vi "Controller.vi"() -> ()   [LabVIEW 2017]
uses:
  <vilib>/Analysis/Matrix/Datatypes/RealMatrix.ctl
  Controls/Force Torque Vector.ctl
  Controls/State.ctl
  Controls/Platform Vectors.ctl
  Controls/Constants.ctl
  Controls/Motor Position.ctl
  <vilib>/Analysis/baseanly.llb/A x Vector.vi
  <vilib>/DAQmx/read.llb/DAQmx Read (Analog 2D DBL NChan NSamp).vi
  <vilib>/Analysis/baseanly.llb/Mean (DBL).vi
  <vilib>/Analysis/baseanly.llb/Real A x B.vi
  <vilib>/Analysis/_algsub.llb/Vector Norm.vi
  <vilib>/Analysis/_algsub.llb/Real Vector Norm.vi
  <vilib>/Analysis/baseanly.llb/Outer Product.vi
  <vilib>/Analysis/baseanly.llb/Real Outer Product.vi
  <vilib>/robotics/Kinematics/Create Lie Group Matrix.vi
  <vilib>/Analysis/7linalg.llb/Create Special Real Matrix.vi
  <vilib>/Analysis/Matrix/Numeric/Multiply/Multiply.vi
  <vilib>/Analysis/Matrix/Numeric/Multiply/Multiply - RM,R.vi
  <vilib>/Analysis/Matrix/Numeric/Multiply/Multiply - R,RM.vi
  <vilib>/Analysis/Matrix/Numeric/Add/Add.vi
  <vilib>/Analysis/Matrix/Numeric/Add/Add - RM,RM.vi
  <vilib>/DAQmx/create/channels.llb/DAQmx Create Channel (AI-Voltage-Basic).vi
  <vilib>/DAQmx/configure/timing.llb/DAQmx Timing (Sample Clock).vi
  <vilib>/DAQmx/miscellaneous.llb/DAQmx Fill In Error Info.vi
  <vilib>/Analysis/3filter.llb/Butterworth Filter (DBL).vi
  <vilib>/Analysis/NI_AALBase.lvlib
  <vilib>/robotics/Kinematics/NI_Kinematics.lvlib
  <vilib>/Analysis/NI_AALPro.lvlib
  <vilib>/Analysis/Matrix/NI_Matrix.lvlib
panel:
  in  "Motor Position":T1
  in  "eta3":dbl=240.0
  in  "eta2":dbl=120.0
  in  "eta1":dbl
  out "dt":dbl=0.017
  in  "gamma2":dbl=72.0
  in  "gamma1":dbl=90.0
  in  "alpha2":dbl=90.0
  in  "alpha1":dbl=90.0
  in  "Constants":T2
  in  "Platform Vectors":T3
  in  "radius":dbl=10.0
  in  "State":T4={"Inertia"=0.5, "Damping"=1.5, "RoM"=0.0}
  out "Waveform Chart":cluster{"Fx":dbl, "Fy":dbl, "Tz":dbl}(graph)={"Fx"=16.845737208367353, "Fy"=-1.0246455882392524, "Tz"=10.011940623114288}
  in  "Force Torque Vector":T5
  in  "Calibration Matrix":T6=[[0.70287, 0.28046, -1.06379, -47.58271, -1.64459, 46.90249], [-0.12905, 55.12684, -1.23322, -27.09022, 0.94146, -27.44249], [69.23154, 1.17633, 67.18151, 0.05352, 69.14468, -0.82584], [0.02366, 0.38743, -1.10802, -0.19684, 1.1351, -0.20033], [1.26658, 0.02633, -0.60731, 0.32903, -0.6386, -0.32248], [0.02624, -0.70869, -0.00313, -0.69424, -0.02408, -0.68399]]
  in  "stop":bool
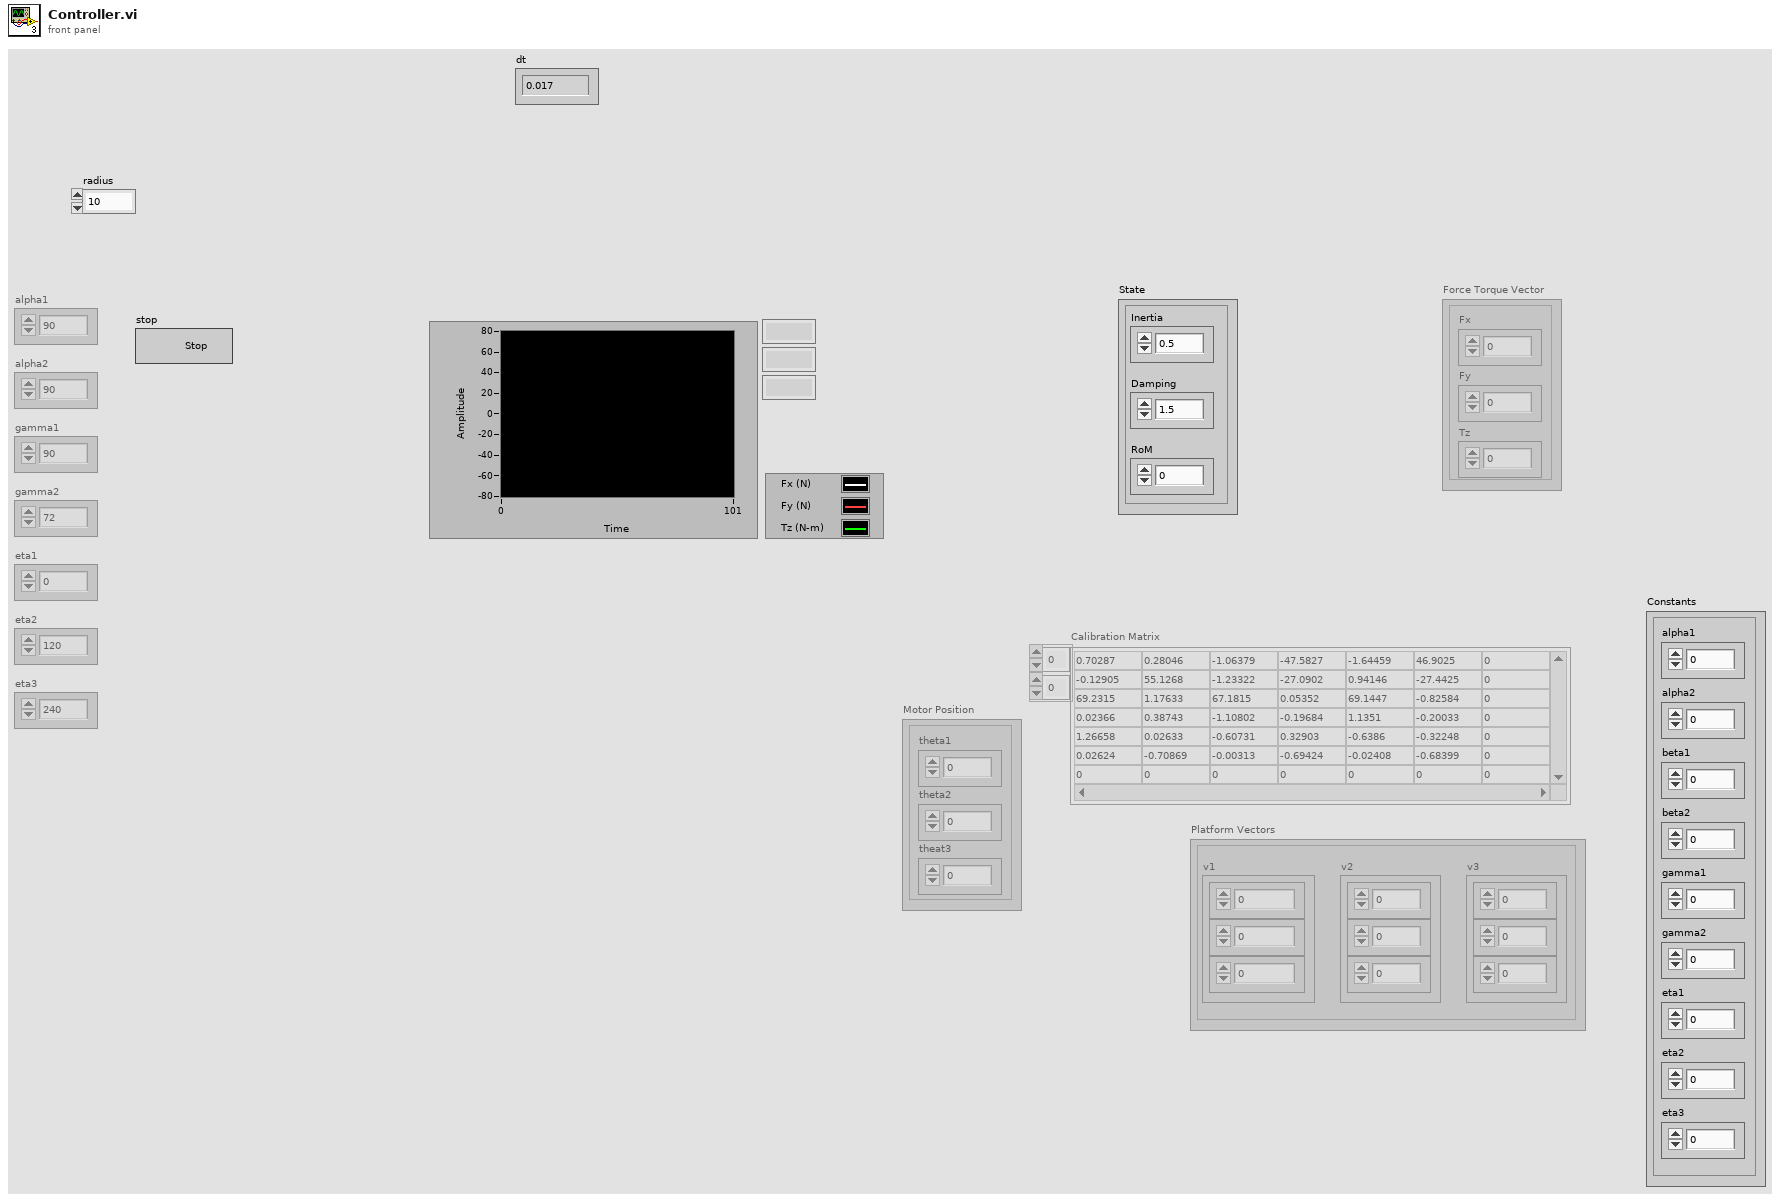
[diagram p1: front panel]
types:
  T1 = typedef "Motor Position.ctl" = cluster{"theta1":dbl, "theta2":dbl, "theat3":dbl}
  T2 = typedef "Constants.ctl" = cluster{"alpha1":dbl, "alpha2":dbl, "beta1":dbl, "beta2":dbl, "gamma1":dbl, "gamma2":dbl, "eta1":dbl, "eta2":dbl, "eta3":dbl}
  T3 = typedef "Platform Vectors.ctl" = cluster{"v1":dbl[], "v2":dbl[], "v3":dbl[]}
  T4 = typedef "State.ctl" = cluster{"Inertia":dbl, "Damping":dbl, "RoM":dbl}
  T5 = typedef "Force Torque Vector.ctl" = cluster{"Fx":dbl, "Fy":dbl, "Tz":dbl}
  T6 = typedef "NI_Matrix.lvlib/RealMatrix.ctl" = dbl[][]
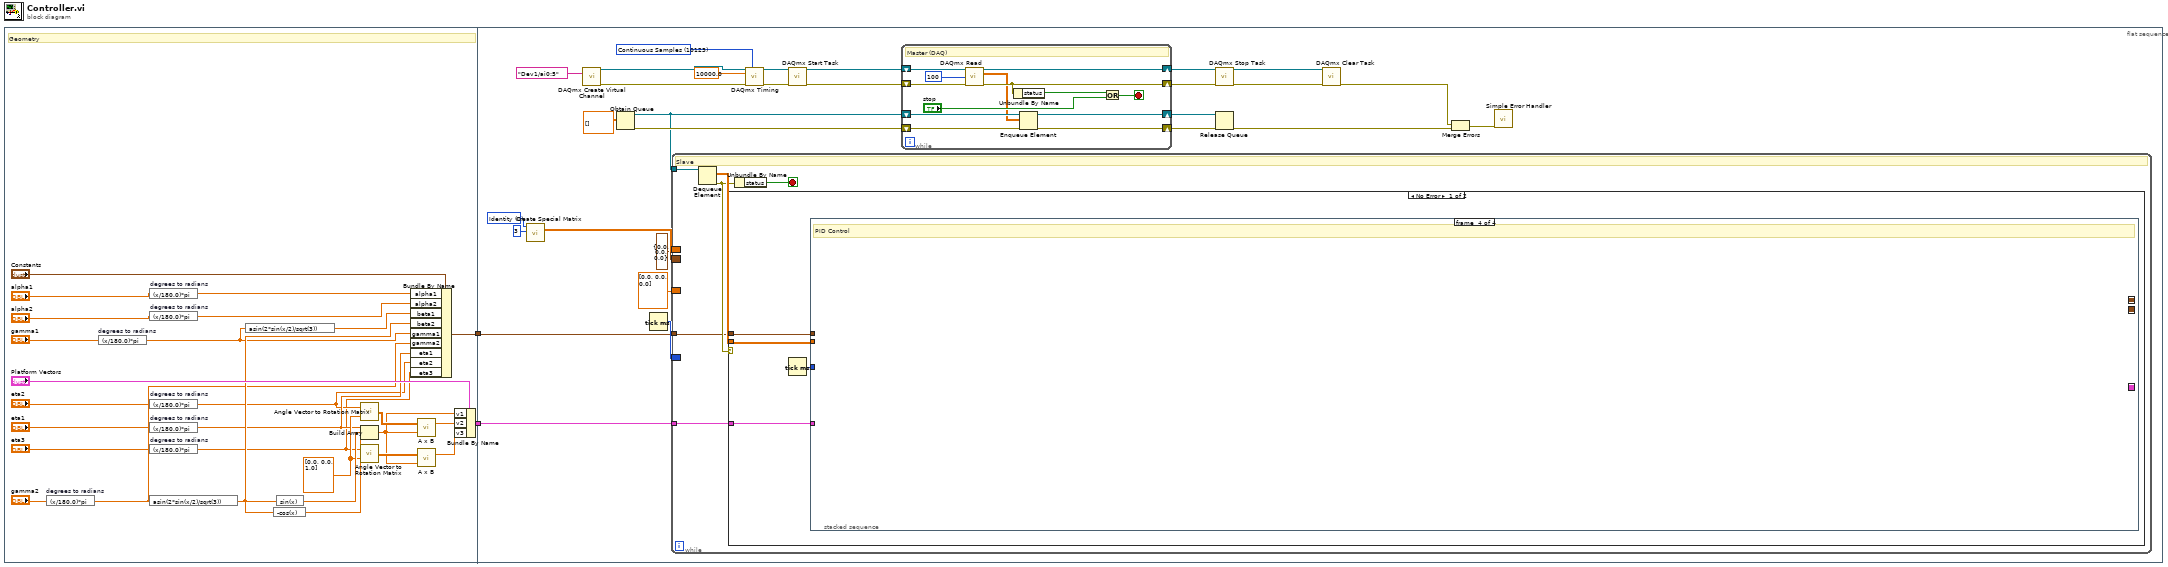
[diagram p0: block diagram]
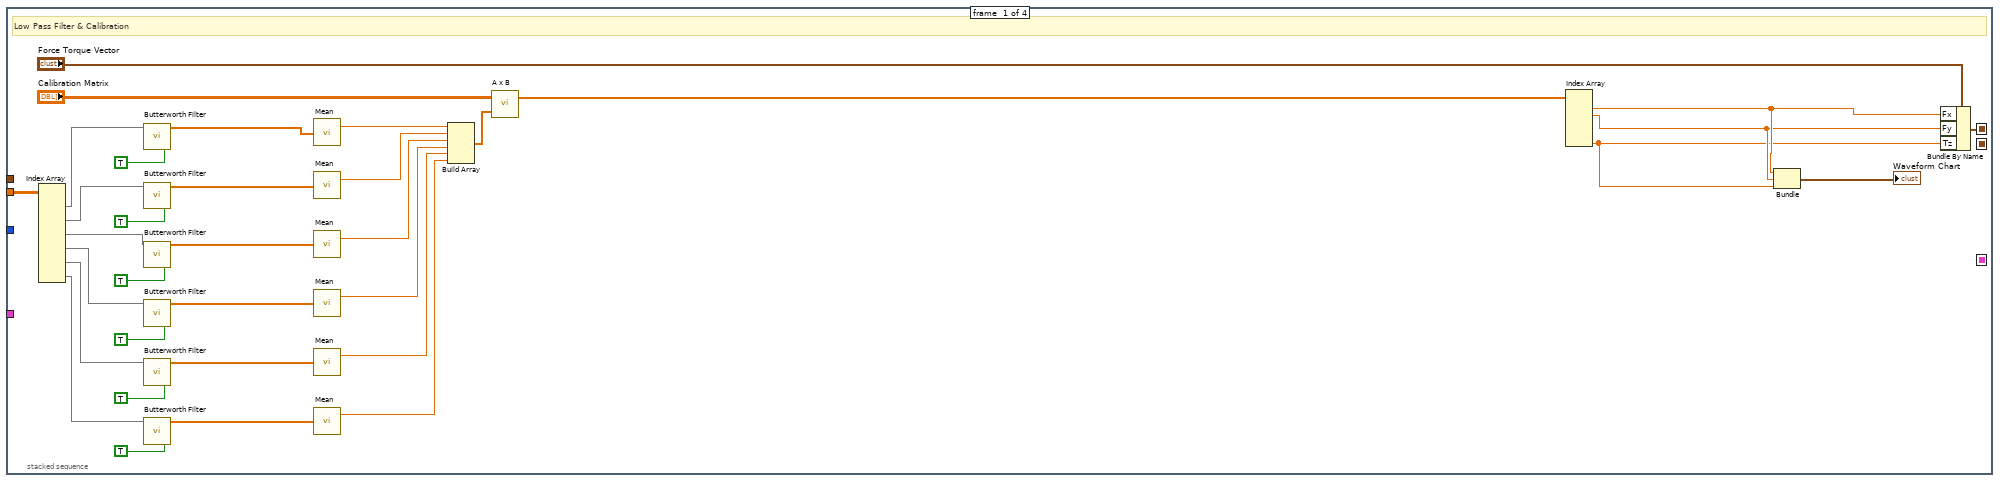
[diagram p2: hidden frame]
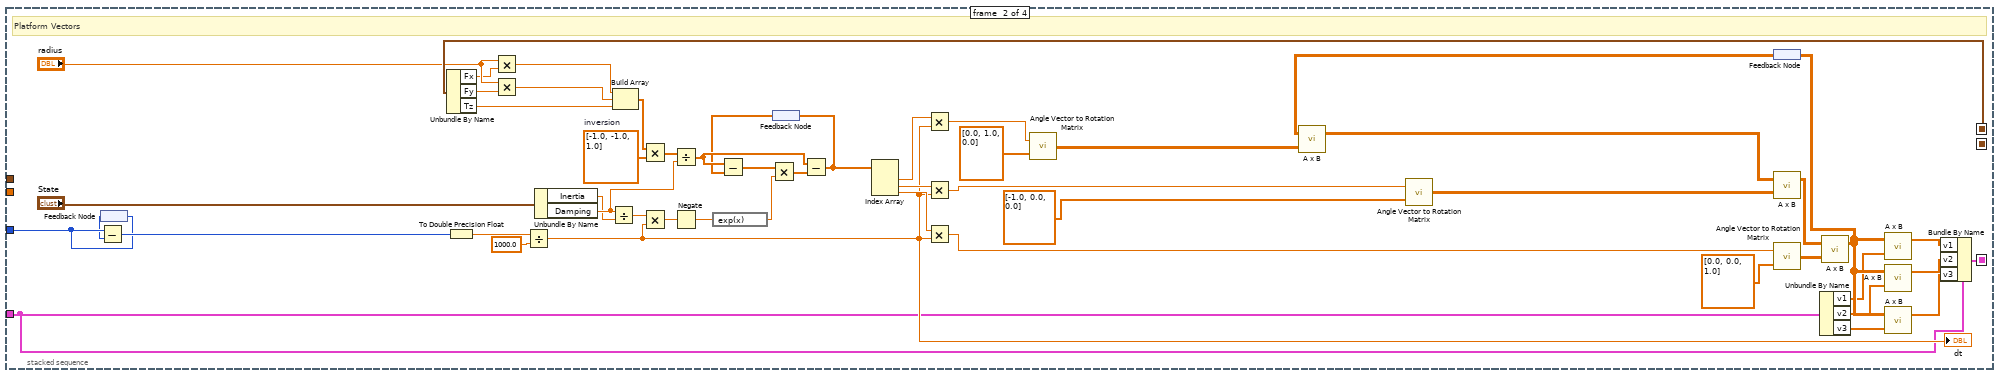
[diagram p3: hidden frame]
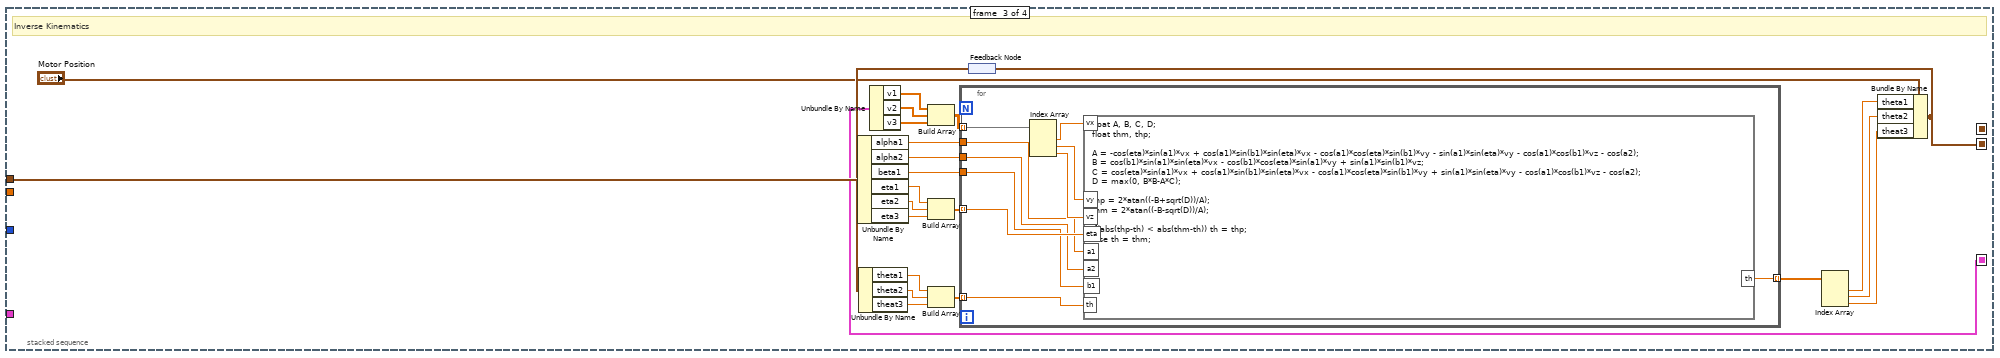
[diagram p4: hidden frame]
diagram:
  n1 = flat-sequence {
    tunnel: [w12] -> w2
    tunnel: [w3] -> w1
    tunnel: w2 -> [w33]
    tunnel: w1 -> [w32]
    frame #0 {
      w17 = dbl[] [0.0, 0.0, 1.0] ("vector")
      # "Geometry"
      n2 = expression code="(x/180.0)*pi" "degrees to radians"("gamma2") -> (w10:dbl)
      n3 = expression code="(x/180.0)*pi" "degrees to radians"("gamma1") -> (w11:dbl)
      n4 = expression code="(x/180.0)*pi" "degrees to radians"("alpha1") -> (w28:dbl)
      n5 = expression code="(x/180.0)*pi" "degrees to radians"("alpha2") -> (w26:dbl)
      n6 = expression code="(x/180.0)*pi" "degrees to radians"("eta2") -> (w5:dbl)
      n7 = expression code="(x/180.0)*pi" "degrees to radians"("eta1") -> (w6:dbl)
      n8 = expression code="(x/180.0)*pi" "degrees to radians"("eta3") -> (w4:dbl)
      n9 = expression code="asin(2*sin(x/2)/sqrt(3))"(w10) -> (w13:dbl)
      n10 = expression code="asin(2*sin(x/2)/sqrt(3))"(w11) -> (w25:dbl)
      n11 = expression code="-cos(x)"(w13) -> (w19:dbl)
      n12 = expression code="sin(x)"(w13) -> (w18:dbl)
      n13 = call <vilib>:"Angle Vector to Rotation Matrix.vi"("vector"=w17, "angle"=w5) -> ("rotation matrix"=w20:T6)
      n14 = Build Array(w6, w18, w19) -> (w16:dbl[])
      n15 = call <vilib>:"Angle Vector to Rotation Matrix.vi"("vector"=w17, "angle"=w4) -> ("rotation matrix"=w21:T6)
      n16 = Bundle By Name(cluster="Constants", "alpha1"=w28, "alpha2"=w26, "beta1"=w25, "beta2"=w13, "gamma1"=w11, "gamma2"=w10, "eta1"=w6, "eta2"=w5, "eta3"=w4) -> (w3:T2)
      n17 = call-poly <vilib>:"A x B.vi"("Vector"=w16, "A"=w20) -> ("A x Vector"=w15:dbl[])  [unwired: 1 out]
      n18 = call-poly <vilib>:"A x B.vi"("Vector"=w16, "A"=w21) -> ("A x Vector"=w14:dbl[])  [unwired: 1 out]
      n19 = Bundle By Name(cluster="Platform Vectors", "v1"=w16, "v2"=w15, "v3"=w14) -> (w12:T3)
    }
    frame #1 {
      w36 = 0 items=["Identity", "Diagonal", "Toeplitz", "Vandermonde", "Companion", "Hankel", "Hadamard", "Wilkinson", "Hilbert", "Inverse Hilbert", "Rosser", "Pascal"] ("matrix type")
      w47 = 10123 items=["Finite Samples"=10178, "Continuous Samples"=10123, "Hardware Timed Single Point"=12522] ("sample mode")
      n20 = call-poly <vilib>:"Create Special Matrix.vi"("matrix type"=w36, "matrix size"=3) -> ("Special Matrix"=w34:T6)  [unwired: 3 in, 1 out]
      n21 = call-poly <vilib>:"DAQmx Create Virtual Channel.vi"("physical channels"=tag "Dev1/ai0:5") -> ("task out"=w58:refnum<k21>, "error out"=w57:errorcluster)  [unwired: 13 in]
      n22 = Obtain Queue(element data type=dbl[][] [] ("data")) -> (queue out=w42:refnum<queue>, error out=w46:errorcluster)  [unwired: 4 in, 1 out]
      n23 = Tick Count (ms)() -> (millisecond timer value=w38:u32)
      n24 = while {
        tunnel: w42 -> [w65]
        border: w38 -> [_]
        border: dbl[] [0.0, 0.0, 0.0] -> [_]
        border: w34 -> [_]
        tunnel: w33 -> [w61]
        tunnel: w32 -> [w60]
        border: T1 {"theta1"=0.0, "theta2"=0.0, "theat3"=0.0} ("Motor Position") -> [_]
        stop <- w64 stop-if-true
        # "Slave"
        n25 = Dequeue Element(queue=w65) -> (element=w63:dbl[][], error out=w62:errorcluster)  [unwired: 2 in, 2 out]
        n26 = case shown="No Error" w62 {
          tunnel: w63 -> [w69 _]
          tunnel: w61 -> [w67 _]
          tunnel: w60 -> [w66 _]
          frame No Error {
            n27 = Tick Count (ms)() -> (millisecond timer value=w68:u32)
            n28 = stacked-sequence {
              seq-local: [w70 _ _ _] -> [_ w131 _ _]
              seq-local: [_ w108 _ _] -> [_ _ w158 _]
              seq-local: [_ _ w156 _] -> [_ _ _ _]
              tunnel: w69 -> [w102 _ _ _]
              tunnel: w68 -> [_ w120 _ _]
              tunnel: w67 -> [_ w107 _ _]
              tunnel: w66 -> [_ _ w175 _]
              frame #0 {
                # "Low Pass Filter & Calibration"
                n29 = Index Array(array=w102) -> (element #1=w103:dbl[], element #2=w101:dbl[], element #3=w100:dbl[], element #4=w99:dbl[], element #5=w98:dbl[], element #6=w97:dbl[])  [unwired: 12 in]
                n30 = call-poly <vilib>:"Butterworth Filter.vi"("init/cont (init:F)"=TRUE, "X"=w103) -> ("Filtered X"=w96:dbl[])  [unwired: 6 in, 1 out]
                n31 = call-poly <vilib>:"Butterworth Filter.vi"("init/cont (init:F)"=TRUE, "X"=w101) -> ("Filtered X"=w95:dbl[])  [unwired: 6 in, 1 out]
                n32 = call-poly <vilib>:"Butterworth Filter.vi"("init/cont (init:F)"=TRUE, "X"=w100) -> ("Filtered X"=w94:dbl[])  [unwired: 6 in, 1 out]
                n33 = call-poly <vilib>:"Butterworth Filter.vi"("init/cont (init:F)"=TRUE, "X"=w99) -> ("Filtered X"=w93:dbl[])  [unwired: 6 in, 1 out]
                n34 = call-poly <vilib>:"Butterworth Filter.vi"("init/cont (init:F)"=TRUE, "X"=w98) -> ("Filtered X"=w92:dbl[])  [unwired: 6 in, 1 out]
                n35 = call-poly <vilib>:"Butterworth Filter.vi"("init/cont (init:F)"=TRUE, "X"=w97) -> ("Filtered X"=w91:dbl[])  [unwired: 6 in, 1 out]
                n36 = call-poly <vilib>:"Mean.vi"("X"=w96) -> ("mean"=w90:dbl)  [unwired: 1 out]
                n37 = call-poly <vilib>:"Mean.vi"("X"=w95) -> ("mean"=w89:dbl)  [unwired: 1 out]
                n38 = call-poly <vilib>:"Mean.vi"("X"=w94) -> ("mean"=w88:dbl)  [unwired: 1 out]
                n39 = call-poly <vilib>:"Mean.vi"("X"=w93) -> ("mean"=w87:dbl)  [unwired: 1 out]
                n40 = call-poly <vilib>:"Mean.vi"("X"=w92) -> ("mean"=w86:dbl)  [unwired: 1 out]
                n41 = call-poly <vilib>:"Mean.vi"("X"=w91) -> ("mean"=w85:dbl)  [unwired: 1 out]
                n42 = Build Array(w90, w89, w88, w87, w86, w85) -> (w76:dbl[])
                n43 = call-poly <vilib>:"A x B.vi"("Vector"=w76, "A"="Calibration Matrix") -> ("A x Vector"=w77:dbl[])  [unwired: 1 out]
                n44 = Index Array(array=w77) -> (element #1=w75:dbl, element #2=w74:dbl, element #6=w73:dbl)  [unwired: 6 in, 3 out]
                n45 = Bundle(w75, w74, w73) -> (→"Waveform Chart":cluster{dbl, dbl, dbl})  [unwired: 1 in]
                n46 = Bundle By Name(cluster="Force Torque Vector", "Fx"=w75, "Fy"=w74, "Tz"=w73) -> (w70:T5)
              }
              frame #1 {
                w105 = dbl[] [-1.0, -1.0, 1.0]  # inversion
                # "Platform Vectors"
                n47 = feedback #1() -> (w119:u32)
                n48 = Subtract(x=w120, y=w119) -> (x-y=w124:u32)
                n49 = feedback-in #1(w120) -> ()
                n50 = Unbundle By Name(w131) -> ("Fx"=w129:dbl, "Fy"=w128:dbl, "Tz"=w125:dbl)
                n51 = To Double Precision Float(number=w124) -> (double precision float=w123:dbl)
                n52 = Multiply(x="radius", y=w129) -> (x*y=w127:dbl)
                n53 = Multiply(x="radius", y=w128) -> (x*y=w126:dbl)
                n54 = Divide(x=w123, y=1000.0) -> (x/y=w121:dbl)
                "dt" <- w121
                n55 = Unbundle By Name("State") -> ("Inertia"=w133:dbl, "Damping"=w134:dbl)
                n56 = Divide(x=w134, y=w133) -> (x/y=w144:dbl)
                n57 = Build Array(w127, w126, w125) -> (w106:dbl[])
                n58 = Multiply(x=w106, y=w105) -> (x*y=w104:dbl[])
                n59 = Multiply(x=w144, y=w121) -> (x*y=w143:dbl)
                n60 = Divide(x=w104, y=w134) -> (x/y=w139:dbl[])
                n61 = Negate(x=w143) -> (-x=w142:dbl)
                n62 = expression code="exp(x)"(w142) -> (w140:dbl)
                n63 = feedback #2() -> (w117:dbl[])
                n64 = Subtract(x=w139, y=w117) -> (x-y=w141:dbl[])
                n65 = Multiply(x=w141, y=w140) -> (x*y=w138:dbl[])
                n66 = Subtract(x=w139, y=w138) -> (x-y=w118:dbl[])
                n67 = feedback-in #2(w118) -> ()
                n68 = Index Array(array=w118) -> (element #1=w136:dbl, element #2=w135:dbl, element #3=w137:dbl)  [unwired: 3 in]
                n69 = Multiply(x=w136, y=w121) -> (x*y=w155:dbl)
                n70 = Multiply(x=w135, y=w121) -> (x*y=w154:dbl)
                n71 = Multiply(x=w137, y=w121) -> (x*y=w153:dbl)
                n72 = call <vilib>:"Angle Vector to Rotation Matrix.vi"("vector"=dbl[] [0.0, 1.0, 0.0], "angle"=w155) -> ("rotation matrix"=w149:T6)
                n73 = call <vilib>:"Angle Vector to Rotation Matrix.vi"("vector"=dbl[] [-1.0, 0.0, 0.0], "angle"=w154) -> ("rotation matrix"=w147:T6)
                n74 = feedback #3() -> (w115:T6)
                n75 = call-poly <vilib>:"A x B.vi"("B"=w149, "A"=w115) -> ("A x B"=w148:T6)  [unwired: 1 out]
                n76 = call-poly <vilib>:"A x B.vi"("B"=w147, "A"=w148) -> ("A x B"=w146:T6)  [unwired: 1 out]
                n77 = call <vilib>:"Angle Vector to Rotation Matrix.vi"("vector"=dbl[] [0.0, 0.0, 1.0], "angle"=w153) -> ("rotation matrix"=w145:T6)
                n78 = Unbundle By Name(w107) -> ("v1"=w114:dbl[], "v2"=w113:dbl[], "v3"=w112:dbl[])
                n79 = call-poly <vilib>:"A x B.vi"("B"=w145, "A"=w146) -> ("A x B"=w116:T6)  [unwired: 1 out]
                n80 = feedback-in #3(w116) -> ()
                n81 = call-poly <vilib>:"A x B.vi"("Vector"=w114, "A"=w116) -> ("A x Vector"=w111:dbl[])  [unwired: 1 out]
                n82 = call-poly <vilib>:"A x B.vi"("Vector"=w113, "A"=w116) -> ("A x Vector"=w110:dbl[])  [unwired: 1 out]
                n83 = call-poly <vilib>:"A x B.vi"("Vector"=w112, "A"=w116) -> ("A x Vector"=w109:dbl[])  [unwired: 1 out]
                n84 = Bundle By Name(cluster=w107, "v1"=w111, "v2"=w110, "v3"=w109) -> (w108:T3)
              }
              frame #2 {
                # "Inverse Kinematics"
                n85 = Unbundle By Name(w175) -> ("alpha1"=w170:dbl, "alpha2"=w169:dbl, "beta1"=w168:dbl, "eta1"=w174:dbl, "eta2"=w173:dbl, "eta3"=w172:dbl)
                n86 = Unbundle By Name(w158) -> ("v1"=w179:dbl[], "v2"=w178:dbl[], "v3"=w177:dbl[])
                n87 = Build Array(w179, w178, w177) -> (w176:dbl[][])
                n88 = Build Array(w174, w173, w172) -> (w171:dbl[])
                n89 = feedback #4() -> (w163:T1)
                n90 = Unbundle By Name(w163) -> ("theta1"=w162:dbl, "theta2"=w161:dbl, "theat3"=w160:dbl)
                n91 = Build Array(w162, w161, w160) -> (w159:dbl[])
                n92 = for {
                  tunnel: w176 -> [w189] mode=indexing
                  tunnel: w171 -> [w185] mode=indexing
                  tunnel: w170 -> [w184]
                  tunnel: w169 -> [w183]
                  tunnel: w168 -> [w182]
                  tunnel: [w181] -> w167 mode=indexing
                  tunnel: w159 -> [w180] mode=indexing
                  n93 = Index Array(array=w189) -> (element #1=w188:dbl, element #2=w187:dbl, element #3=w186:dbl)  [unwired: 3 in]
                  n94 = formula code="float A, B, C, D;\nfloat thm, thp;\n\nA = -cos(eta)*sin(a1)*vx + cos(a1)*sin(b1)*sin(eta)*vx - cos(a1)*cos(eta)*sin(b1)*vy - sin(a1)*sin(eta)*vy - cos(a1)*cos(b1)*vz - cos(a2);\nB = cos(b1)*sin(a1)*sin(eta)*vx - cos(b1)*cos(eta)*sin(a1)*vy + sin(a1)*sin(b1)*vz;\nC = cos(eta)*sin(a1)*vx + cos(a1)*sin(b1)*sin(eta)*vx - cos(a1)*cos(eta)*sin(b1)*vy + sin(a1)*sin(eta)*vy - cos(a1)*cos(b1)*vz - cos(a2);\nD = max(0, B*B-A*C);\n\nthp = 2*atan((-B+sqrt(D))/A); \nthm = 2*atan((-B-sqrt(D))/A); \n\nif(abs(thp-th) < abs(thm-th)) th = thp;\nelse th = thm;"("vx"=w188, "vy"=w187, "vz"=w186, "eta"=w185, "a1"=w184, "b1"=w182, "a2"=w183, "th"=w180) -> ("th"=w181:dbl)
                }
                n95 = Index Array(array=w167) -> (element #1=w166:dbl, element #2=w165:dbl, element #3=w164:dbl)  [unwired: 3 in]
                n96 = Bundle By Name(cluster="Motor Position", "theta1"=w166, "theta2"=w165, "theat3"=w164) -> (w156:T1)
                n97 = feedback-in #4(w156) -> ()
              }
              frame #3 {
                # "PID Control"
              }
            }
          }
          frame Error {
          }
        }
        n98 = Unbundle By Name(w62) -> ("status"=w64:bool)
      }
      n99 = call-poly <vilib>:"DAQmx Timing.vi"("task/channels in"=w58, "sample mode"=w47, "rate"=10000.0, "error in"=w57) -> ("task out"=w55:refnum<k21>, "error out"=w56:errorcluster)  [unwired: 10 in]
      n100 = call <vilib>:"DAQmx Start Task.vi"("task/channels in"=w55, "error in"=w56) -> ("task out"=w54:refnum<k21>, "error out"=w51:errorcluster)  [unwired: 12 in]
      n101 = while {
        shift-right: [w193] -> w41
        shift-left: w42 -> [w194]
        shift-right: [w191] -> w40
        shift-left: w46 -> [w192]
        shift-right: [w201] -> w53
        shift-left: w54 -> [w202]
        shift-right: [w198] -> w50
        shift-left: w51 -> [w200]
        stop <- w195 stop-if-true
        # "Master (DAQ)"
        n102 = call-poly <vilib>:"DAQmx Read.vi"("task/channels in"=w202, "number of samples per channel"=100, "error in"=w200) -> ("task out"=w201:refnum<k21>, "data"=w190:dbl[][], "error out"=w198:errorcluster)  [unwired: 10 in]
        n103 = Unbundle By Name(w198) -> ("status"=w197:bool)
        n104 = Enqueue Element(queue=w194, element=w190, error in (no error)=w192) -> (queue out=w193:refnum<queue>, error out=w191:errorcluster)  [unwired: 1 in, 1 out]
        n105 = Or(x=w197, y="stop") -> (x .or. y?=w195:bool)
      }
      n106 = call <vilib>:"DAQmx Stop Task.vi"("task/channels in"=w53, "error in"=w50) -> ("task out"=w52:refnum<k21>, "error out"=w49:errorcluster)  [unwired: 12 in]
      n107 = Release Queue(queue=w41, error in (no error)=w40) -> (error out=w39:errorcluster)  [unwired: 1 in, 2 out]
      n108 = call <vilib>:"DAQmx Clear Task.vi"("task in"=w52, "error in"=w49) -> ("error out"=w44:errorcluster)  [unwired: 13 in]
      n109 = Merge Errors(w44, w39) -> (w45:errorcluster)
      n110 = call <vilib>:"Simple Error Handler.vi"("error in (no error)"=w45) -> ()  [unwired: 4 in, 5 out]
    }
  }
